vi "Read visible.vi"(8 "error in (no error)":errorcluster, 11 "TextDecoration in":refnum<class "TextDecoration.lvclass">) -> (0 "error out":errorcluster, 2 "visible":bool, 3 "TextDecoration out":refnum<class "TextDecoration.lvclass">)   [LabVIEW 2023, in "TLC_Scripto.lvlib" / "TextDecoration.lvclass"]
uses:
  TextDecoration.lvclass
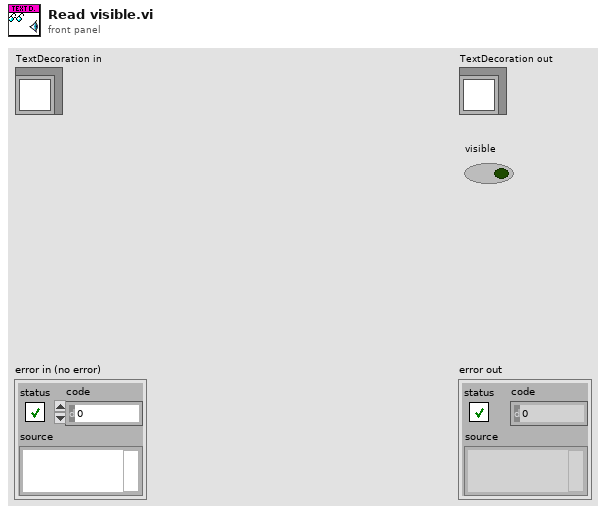
[diagram p1: front panel]
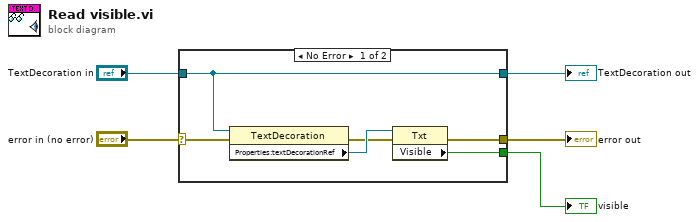
[diagram p0: block diagram]
diagram:
  n1 = case shown="No Error" "error in (no error)" {
    selector: "error in (no error)" -> [w8 w12]
    tunnel: [w7 w12] -> w4
    tunnel: [w9 w13] -> w2
    tunnel: "TextDecoration in" -> [w9 w13]
    tunnel: [w6 _] -> w1
    frame No Error {
      n2 = property class="TextDecoration"(reference=w9, error in=w8) -> (error out=w10:errorcluster, "Properties:textDecorationRef"=w11:refnum<vi>)  [unwired: 1 out]
      n3 = property class="Txt"(reference=w11, error in=w10) -> (error out=w7:errorcluster, "Visible"=w6:bool)  [unwired: 1 out]
    }
    frame Error {
    }
  }
  "error out" <- w4
  "TextDecoration out" <- w2
  "visible" <- w1
